vi "Find Corrupted Distance.vi"() -> ()   [LabVIEW 2016]
panel:
  out "b1":dbl
  in  "x":dbl
  in  "beta(in deg)":dbl
  in  "b2":dbl
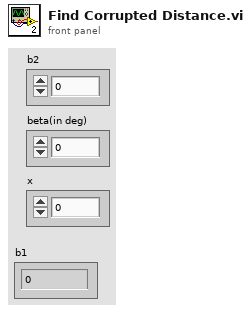
[diagram p1: front panel]
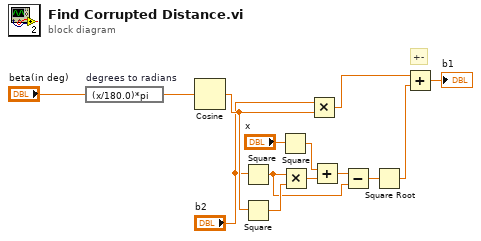
[diagram p0: block diagram]
diagram:
  # "+-"
  n1 = expression code="(x/180.0)*pi" "degrees to radians"("beta(in deg)") -> (w13:dbl)
  n2 = Cosine(x=w13) -> (cos(x)=w3:dbl)
  n3 = Square(x="b2") -> (x^2=w1:dbl)
  n4 = Square(x=w3) -> (x^2=w12:dbl)
  n5 = Square(x="x") -> (x^2=w9:dbl)
  n6 = Multiply(x=w1, y=w12) -> (x*y=w11:dbl)
  n7 = Multiply(x="b2", y=w3) -> (x*y=w4:dbl)
  n8 = Add(x=w9, y=w11) -> (x+y=w8:dbl)
  n9 = Subtract(x=w8, y=w1) -> (x-y=w7:dbl)
  n10 = Square Root(x=w7) -> (sqrt(x)=w6:dbl)
  n11 = Add(x=w4, y=w6) -> (x+y=→"b1":dbl)
